vi "New.vi"(8 "error in (no error)":errorcluster, 10 "timeout":i32=10000, 11 "Socket.Base in":refnum<class "Socket.Base.lvclass">) -> (0 "error out":errorcluster, 3 "Socket.Base out":refnum<class "Socket.Base.lvclass">)   [LabVIEW 2014, in "Socket.lvlib" / "Socket.Base.lvclass"]
doc: "Creates a new socket object. Must be run to set the timeout and the \"initialized\" property"
uses:
  Socket.Base.lvclass
  Socket.Base.lvclass/Socket.Base.ctl
  Accessors/Write timeout.vi
  Accessors/Write connected.vi
  Accessors/Write initialized.vi
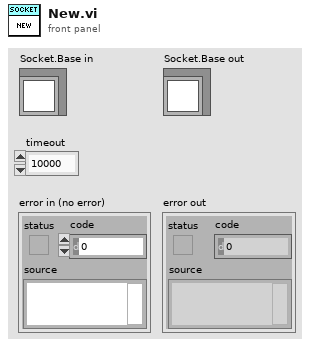
[diagram p1: front panel]
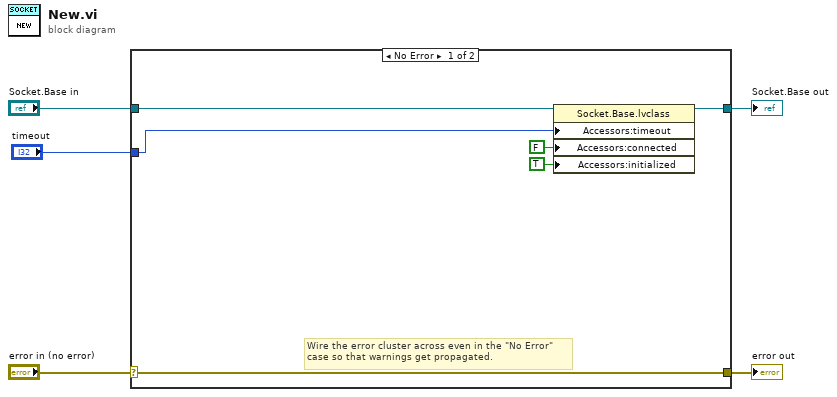
[diagram p0: block diagram]
diagram:
  n1 = case shown="No Error" "error in (no error)" {
    selector: "error in (no error)" -> [w11 w13]
    tunnel: [w11 w13] -> w4
    tunnel: [w9 w12] -> w2
    tunnel: "Socket.Base in" -> [w10 w12]
    tunnel: "timeout" -> [w8 _]
    frame No Error {
      # "Wire the error cluster across even in the \"No Error\"\ncase so that warnings get propagated."
      n2 = property class="Socket.Base.lvclass"(reference=w10, "Accessors:timeout"=w8, "Accessors:connected"=FALSE ("connected"), "Accessors:initialized"=TRUE ("initialized")) -> (reference out=w9:refnum<class "Socket.Base.lvclass">)  [unwired: 1 in, 1 out]
    }
    frame Error {
    }
  }
  "error out" <- w4
  "Socket.Base out" <- w2
